vi "MGI VI Tree.vi"(11 "MGI Error Reporter Dialog.lvclass":refnum<class "MGI Error Reporter Dialog.lvclass">) -> ()   [LabVIEW 2020, in "MGI Error Reporter Dialog.lvclass"]
doc: "This VI documents the MGI Error Reporter Dialog Class.\nSee Block Diagram for documentation.\n\nAuthored by Shawn Walpole\nsupport@mooregoodideas.com\nwww.mooregoodideas.com\n\nCopyright (c) 2013, Moore Good Ideas, Inc.\n\nAll rights reserved.\n\nRedistribution and use in source and binary forms, with or without modification, are permitted provided that the following conditions are met:\n\n * Redistributions of source code must retain the above copyright notice, this list of conditions and the following disclaimer.\n * Redistributions in binary form must reproduce the above copyright notice, this list of conditions and the following disclaimer in the documentation and/or other materials provided with the distribution.\n * Neither the name of Moore Good Ideas, Inc. nor the names of its contributors may be used to endorse or promote products derived from this software without specific prior written permission.\n\nTHIS SOFTWARE IS PROVIDED BY THE COPYRIGHT HOLDERS AND CONTRIBUTORS \"AS IS\" AND ANY EXPRESS OR IMPLIED WARRANTIES, INCLUDING, BUT NOT LIMITED TO, THE IMPLIED WARRANTIES OF MERCHANTABILITY AND FITNESS FOR A PARTICULAR PURPOSE ARE DISCLAIMED. IN NO EVENT SHALL THE COPYRIGHT OWNER OR CONTRIBUTORS BE LIABLE FOR ANY DIRECT, INDIRECT, INCIDENTAL, SPECIAL, EXEMPLARY, OR CONSEQUENTIAL DAMAGES (INCLUDING, BUT NOT LIMITED TO, PROCUREMENT OF SUBSTITUTE GOODS OR SERVICES; LOSS OF USE, DATA, OR PROFITS; OR BUSINESS INTERRUPTION) HOWEVER CAUSED AND ON ANY THEORY OF LIABILITY, WHETHER IN CONTRACT, STRICT LIABILITY, OR TORT (INCLUDING NEGLIGENCE OR OTHERWISE) ARISING IN ANY WAY OUT OF THE USE OF THIS SOFTWARE, EVEN IF ADVISED OF THE POSSIBILITY OF SUCH DAMAGE."
uses:
  <userlib>/_MGI/Error Reporter/MGI Error Reporter Dialog/MGI Error Reporter Dialog.lvclass
  <userlib>/_MGI/Error Reporter/MGI Error Reporter Dialog/Protected/MGI Dialog UI Refs Cluster.ctl
  <userlib>/_MGI/Error Reporter/MGI Error Reporter Dialog/Protected/MGI Control Enum.ctl
  <userlib>/_MGI/Error Reporter/MGI Error Reporter Dialog/MGI ERD LB Row Time and Count/MGI ERD LB Row Time and Count.lvclass
  <userlib>/_MGI/Error Reporter/MGI Error Reporter Dialog/MGI ERD LB Row Base/MGI ERD LB Row Base.lvclass
  <userlib>/_MGI/Error Reporter/MGI Error Reporter Base/MGI Error Reporter Base.lvclass
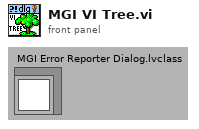
[diagram p1: front panel]
types:
  T1 = typedef "MGI Error Reporter Dialog.lvclass/MGI Control Enum.ctl" = enum16{"Error LB", "Details String", "Caller Ring", "Message String", "Clear Button"}
  T2 = typedef "MGI Error Reporter Dialog.lvclass/MGI Dialog UI Refs Cluster.ctl" = cluster{"LB Ref":refnum<vi>, "Details Ref":refnum<vi>, "Caller Ring Ref":refnum<vi>, "Message Ref":refnum<vi>, "Clear Btn Ref":refnum<vi>}
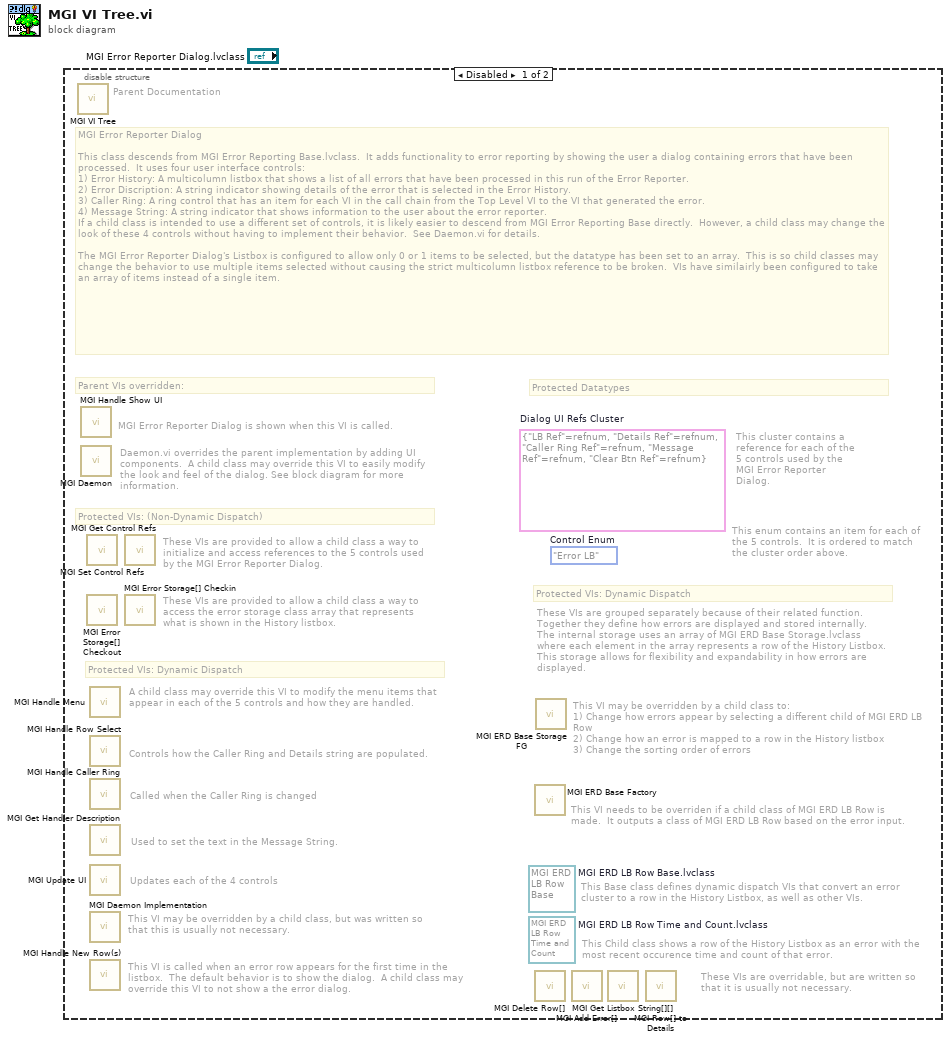
[diagram p0: block diagram]
diagram:
  n1 = disable-structure shown="Disabled" {
    frame Disabled {
      (unwired) refnum<class "MGI ERD LB Row Base.lvclass"> refnum  # MGI ERD LB Row Base.lvclass
      (unwired) refnum<class "MGI ERD LB Row Time and Count.lvclass"> refnum  # MGI ERD LB Row Time and Count.lvclass
      (unwired) MGI_Control_Enum."Error LB"  # Control Enum
      (unwired) T2 {"LB Ref"=refnum, "Details Ref"=refnum, "Caller Ring Ref"=refnum, "Message Ref"=refnum, "Clear Btn Ref"=refnum}  # Dialog UI Refs Cluster
      # "This VI is called when an error row appears for the first time in the listbox.  The default behavior is to show the dialog.  A child class may override this VI to not show a the error dialog."
      # "This VI needs to be overriden if a child class of MGI ERD LB Row is made.  It outputs a class of MGI ERD LB Row based on the error input."
      # "Called when the Caller Ring is changed"
      # "This Child class shows a row of the History Listbox as an error with the most recent occurence time and count of that error."
      # "This Base class defines dynamic dispatch VIs that convert an error cluster to a row in the History Listbox, as well as other VIs."
      # "These VIs are provided to allow a child class a way to access the error storage class array that represents what is shown in the History listbox."
      # "This VI may be overridden by a child class to:\n1) Change how errors appear by selecting a different child of MGI ERD LB Row\n2) Change how an error is mapped to a row in the History listbox\n3) Change the sorting order of errors"
      # "Used to set the text in the Message String."
      # "Updates each of the 4 controls"
      # "Controls how the Caller Ring and Details string are populated."
      # "A child class may override this VI to modify the menu items that appear in each of the 5 controls and how they are handled."
      # "This VI may be overridden by a child class, but was written so that this is usually not necessary."
      # "These VIs are overridable, but are written so that it is usually not necessary."
      # "These VIs are grouped separately because of their related function.  Together they define how errors are displayed and stored internally.\nThe internal storage uses an array of MGI ERD Base Storage.lvclass where each element in the array represents a row of the History Listbox.  This storage allows for flexibility and expandability in how errors are displayed."
      # "Protected VIs: Dynamic Dispatch"
      # "These VIs are provided to allow a child class a way to initialize and access references to the 5 controls used by the MGI Error Reporter Dialog."
      # "Daemon.vi overrides the parent implementation by adding UI components.  A child class may override this VI to easily modify the look and feel of the dialog. See block diagram for more information."
      # "MGI Error Reporter Dialog is shown when this VI is called."
      # "Parent VIs overridden:"
      # "This enum contains an item for each of the 5 controls.  It is ordered to match the cluster order above."
      # "This cluster contains a reference for each of the 5 controls used by the MGI Error Reporter Dialog."
      # "Protected Datatypes"
      # "Protected VIs: (Non-Dynamic Dispatch)"
      # "Protected VIs: Dynamic Dispatch"
      # "Parent Documentation"
      # "MGI Error Reporter Dialog\n\nThis class descends from MGI Error Reporting Base.lvclass.  It adds functionality to error reporting by showing the user a dialog containing errors that have been processed.  It uses four user interface controls:\n1) Error History: A multicolumn listbox that shows a list of all errors that have been processed in this run of the Error Reporter.\n2) Error Discription: A string indicator showing details of the error that is selected in the Error History.\n3) Caller Ring: A ring control that has an item for each VI in the call chain from the Top Level VI to the VI that generated the error.\n4) Message String: A string indicator that shows information to the user about the error reporter.\nIf a child class is intended to use a different set of controls, it is likely easier to descend from MGI Error Reporting Base directly.  However, a child class may change the look of these 4 controls without having to implement their behavior.  See Daemon.vi for details.\n\nThe MGI Error Reporter Dialog's Listbox is configured to allow only 0 or 1 items to be selected, but the datatype has been set to an array.  This is so child classes may change the behavior to use multiple items selected without causing the strict multicolumn listbox reference to be broken.  VIs have similairly been configured to take an array of items instead of a single item."
      n2 = call-parent "MGI VI Tree.vi"() -> ()  [unwired: 12 in]
      n3 = call-dynamic "MGI Handle Show UI.vi"() -> ()  [unwired: 10 in, 2 out]
      n4 = call-dynamic "MGI Daemon.vi"() -> ()  [unwired: 11 in, 1 out]
      n5 = call <userlib>:"MGI Set Control Refs.vi"() -> ()  [unwired: 11 in, 1 out]
      n6 = call <userlib>:"MGI Error Storage[] Checkout.vi"() -> ()  [unwired: 10 in, 2 out]
      n7 = call-dynamic "MGI Handle Menu.vi"() -> ()  [unwired: 9 in, 3 out]
      n8 = call-dynamic "MGI Handle Row Select.vi"() -> ()  [unwired: 10 in, 2 out]
      n9 = call-dynamic "MGI Handle Caller Ring.vi"() -> ()  [unwired: 10 in, 2 out]
      n10 = call-dynamic "MGI Get Handler Description.vi"() -> ()  [unwired: 10 in, 2 out]
      n11 = call-dynamic "MGI Update UI.vi"() -> ()  [unwired: 10 in, 2 out]
      n12 = call-dynamic "MGI Daemon Implementation.vi"() -> ()  [unwired: 11 in, 1 out]
      n13 = call-dynamic "MGI Handle New Row(s).vi"() -> ()  [unwired: 10 in, 2 out]
      n14 = call <userlib>:"MGI Get Control Refs.vi"() -> ()  [unwired: 11 in, 1 out]
      n15 = call <userlib>:"MGI Error Storage[] Checkin.vi"() -> ()  [unwired: 11 in, 1 out]
      n16 = call-dynamic "MGI ERD Base Factory.vi"() -> ()  [unwired: 11 in, 1 out]
      n17 = call-dynamic "MGI Delete Row[].vi"() -> ()  [unwired: 10 in, 2 out]
      n18 = call-dynamic "MGI ERD Base Storage FG.vi"() -> ()  [unwired: 10 in, 2 out]
      n19 = call-dynamic "MGI Add Error[].vi"() -> ()  [unwired: 10 in, 2 out]
      n20 = call-dynamic "MGI Get Listbox String[][].vi"() -> ()  [unwired: 10 in, 2 out]
      n21 = call-dynamic "MGI Row[] to Details.vi"() -> ()  [unwired: 9 in, 3 out]
    }
    frame Enabled {
    }
  }
